vi "Wait until VIs close.vi"(8 "error in (no error)":errorcluster, 10 "Timeout (s)":dbl=-1.0 format="%#_13g", 11 "VI Ref In[]":refnum<vi>[](array[refnum])) -> (0 "error out":errorcluster, 2 "Timed Out?":bool, 3 "VI Ref Out[]":refnum<vi>[](array[refnum]))   [LabVIEW 2016, in "SLL Application.lvlib"]
doc: "Waits for either all VIs wired in the input (as reference) to close, or the specified timeout occurs, whichever is earlier.\nThis VI runs normally even if an error occurred before this VI."
uses:
  SLL Application.lvlib
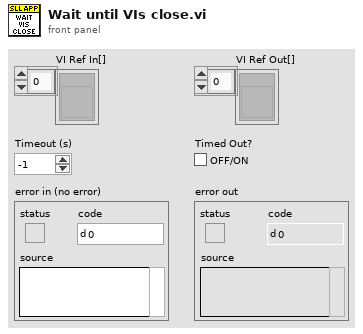
[diagram p1: front panel]
types:
  T1 = enum32{"Bad", "Idle", "Run top level", "Running"}
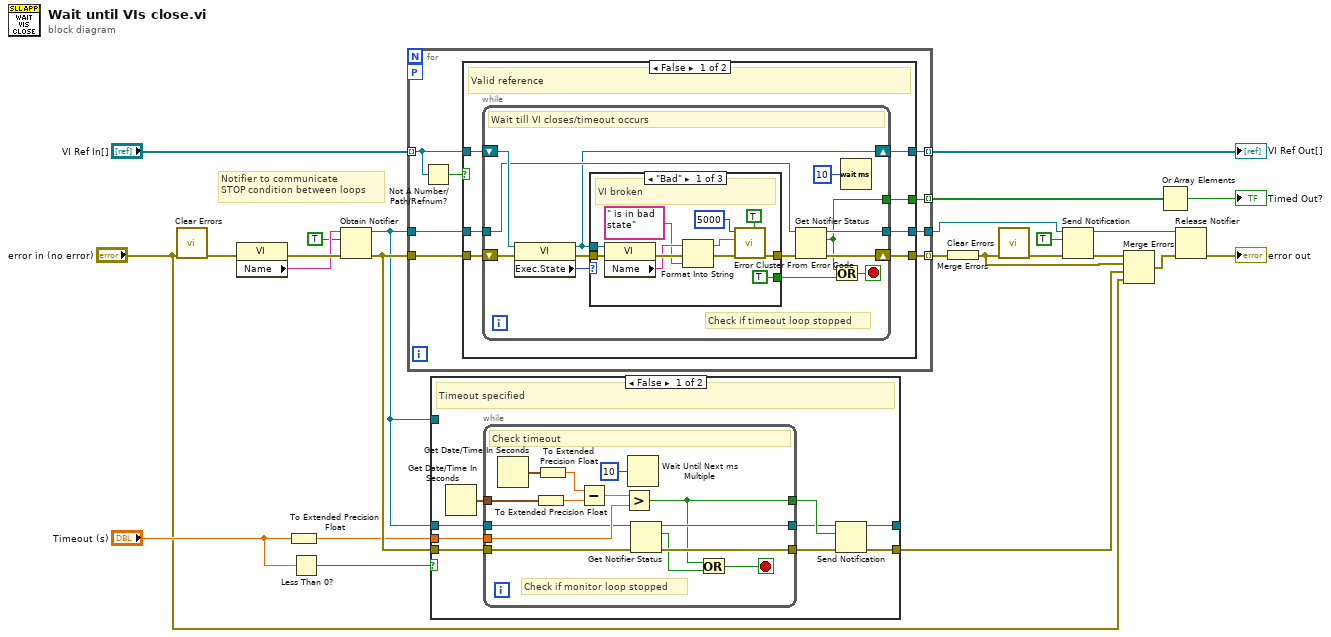
[diagram p0: block diagram]
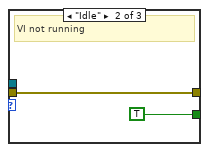
[diagram p2: hidden frame]
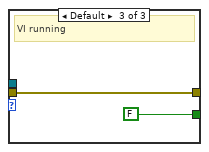
[diagram p3: hidden frame]
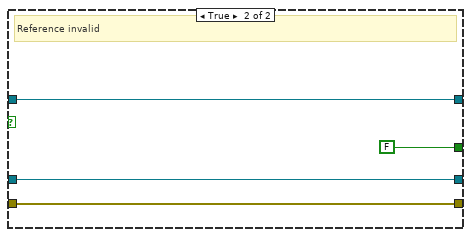
[diagram p4: hidden frame]
diagram:
  # "Notifier to communicate \nSTOP condition between loops"
  n1 = call <vilib>:"Clear Errors.vi"("error in (no error)"="error in (no error)") -> ("error out"=w12:errorcluster)  [unwired: 5 in, 1 out]
  n2 = property class="VI"(error in=w12) -> (error out=w20:errorcluster, "Name"=w19:string)  [unwired: 1 in, 1 out]
  n3 = To Extended Precision Float(1:"Timeout (s)") -> (0:w13:ext)
  n4 = Less Than 0?(x="Timeout (s)") -> (x < 0?=w14:bool)
  n5 = Obtain Notifier(name (unnamed)=w19, notification data type=TRUE, error in (no error)=w20) -> (notifier out=w8:refnum<notifier>, error out=w21:errorcluster)  [unwired: 1 in, 1 out]
  n6 = for {
    tunnel: "VI Ref In[]" -> [w31] mode=indexing
    workers-P: _ -> [_]
    tunnel: w21 -> [w30]
    tunnel: [w29] -> w23 mode=indexing
    tunnel: [w28] -> w22 mode=indexing
    tunnel: w8 -> [w27]
    tunnel: [w26] -> w10
    tunnel: [w25] -> w16 mode=indexing
    n7 = Not A Number/Path/Refnum?(number/path/refnum=w31) -> (NaN/Path/Refnum?=w32:bool)
    n8 = case shown="False" w32 {
      tunnel: w31 -> [w39 w70]
      tunnel: w30 -> [w38 w71]
      tunnel: [w37 w71] -> w29
      tunnel: [w36 w70] -> w28
      tunnel: w27 -> [w35 w68]
      tunnel: [w34 w68] -> w26
      tunnel: [w33 FALSE] -> w25
      frame False {
        # "Valid reference"
        n9 = while {
          shift-right: [w40] -> w36
          shift-left: w39 -> [w51]
          shift-right: [w45] -> w37
          shift-left: w38 -> [w52]
          tunnel: w35 -> [w46]
          tunnel: [w43] -> w34
          tunnel: [w41] -> w33
          stop <- w42 stop-if-true
          # "Check if timeout loop stopped"
          # "Wait till VI closes/timeout occurs"
          n10 = property class="VI"(reference=w51, error in=w52) -> (reference out=w40:refnum<vi>, error out=w48:errorcluster, "Exec.State"=w50:T1)
          n11 = case shown="\"Bad\"" w50 {
            tunnel: [TRUE TRUE FALSE] -> w49
            tunnel: [w63 w64 w66] -> w44
            tunnel: w48 -> [w58 w64 w66]
            tunnel: w40 -> [w59 _ _]
            frame "Bad" {
              # "VI broken"
              n12 = property class="VI"(reference=w59, error in=w58) -> (error out=w57:errorcluster, "Name"=w55:string)  [unwired: 1 out]
              n13 = Format Into String(initial string=w55, error in=w57, " is in bad state" ("error message (\"\")")) -> (resulting string=w53:string, error out=w56:errorcluster)  [unwired: 1 in]
              n14 = call <vilib>:"Error Cluster From Error Code.vi"("is warning? (False)"=TRUE, "error in (no error)"=w56, "error message (\"\")"=w53, "error code (0)"=5000) -> ("error out"=w63:errorcluster)  [unwired: 5 in]
            }
            frame "Idle" {
              # "VI not running"
            }
            frame Default {
              # "VI running"
            }
          }
          n15 = Get Notifier Status(notifier=w46, error in (no error)=w44) -> (notifier out=w43:refnum<notifier>, current notification=w41:bool, error out=w45:errorcluster)  [unwired: 2 out]
          n16 = Or(x=w41, y=w49) -> (x .or. y?=w42:bool)
          n17 = Wait (ms)(milliseconds to wait=u32 10) -> ()  [unwired: 1 out]
        }
      }
      frame True {
        # "Reference invalid"
      }
    }
  }
  "VI Ref Out[]" <- w22
  n18 = case shown="False" w14 {
    tunnel: w13 -> [w79 _]
    tunnel: w8 -> [_ w95]
    tunnel: w21 -> [w78 w96]
    tunnel: [w76 w96] -> w3
    tunnel: [w75 w95] -> _
    tunnel: w8 -> [w73 _]
    frame False {
      # "Timeout specified"
      n19 = Get Date/Time In Seconds() -> (seconds since 1Jan1904=w80:timestamp)
      n20 = while {
        tunnel: w80 -> [w94]
        tunnel: w79 -> [w88]
        tunnel: [w83] -> w74
        tunnel: w78 -> [w87]
        tunnel: [w86] -> w77
        tunnel: w73 -> [w85]
        tunnel: [w84] -> w72
        stop <- w81 stop-if-true
        # "Check if monitor loop stopped"
        # "Check timeout"
        n21 = Get Date/Time In Seconds() -> (seconds since 1Jan1904=w93:timestamp)
        n22 = To Extended Precision Float(1:w94) -> (0:w92:ext)
        n23 = To Extended Precision Float(1:w93) -> (0:w91:ext)
        n24 = Subtract(x=w91, y=w92) -> (x-y=w89:ext)
        n25 = Greater?(x=w89, y=w88) -> (0:w83:bool)
        n26 = Wait Until Next ms Multiple(millisecond multiple=u32 10) -> ()  [unwired: 1 out]
        n27 = Get Notifier Status(notifier=w85, error in (no error)=w87) -> (notifier out=w84:refnum<notifier>, current notification=w82:bool, error out=w86:errorcluster)  [unwired: 2 out]
        n28 = Or(x=w83, y=w82) -> (x .or. y?=w81:bool)
      }
      n29 = Send Notification(notification=w74, notifier=w72, error in (no error)=w77) -> (notifier out=w75:refnum<notifier>, error out=w76:errorcluster)
    }
    frame True {
      # "Timeout not specified"
    }
  }
  n30 = Merge Errors(w23) -> (w1:errorcluster)
  n31 = call <vilib>:"Clear Errors.vi"("error in (no error)"=w1) -> ("error out"=w2:errorcluster)  [unwired: 5 in, 1 out]
  n32 = Send Notification(notification=TRUE, notifier=w10, error in (no error)=w2) -> (notifier out=w4:refnum<notifier>, error out=w7:errorcluster)
  n33 = Merge Errors(w7, w1, w3, "error in (no error)") -> (w6:errorcluster)
  n34 = Or Array Elements(Boolean array=w16) -> (logical OR=→"Timed Out?":bool)
  n35 = Release Notifier(notifier=w4, error in (no error)=w6) -> (error out=→"error out":errorcluster)  [unwired: 1 in, 2 out]
